vi "Add Item Buffered.vi"(6 "Items Array Length":i32=5, 8 "错误输入":errorcluster, 10 "Item":string, 11 "Listbox Ref":refnum<vi>) -> (0 "错误输出":errorcluster, 3 "Dup Listbox Ref":refnum<vi>)   [LabVIEW 2012, in "Listbox Tool.lvlib"]
uses:
  Listbox Tool.lvlib
  Custom Type/Read and Write Mode.ctl
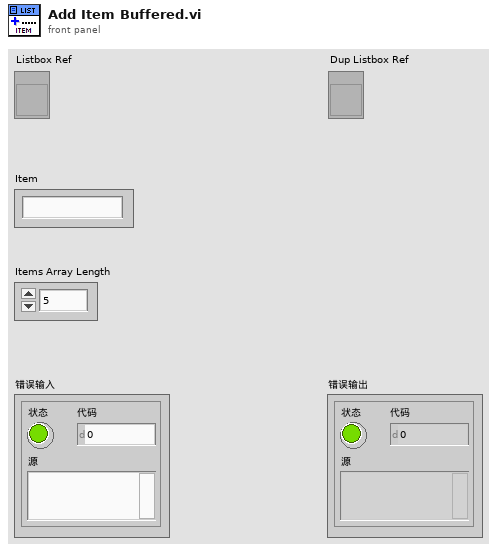
[diagram p1: front panel]
types:
  T1 = typedef "Listbox Tool.lvlib/Read and Write Mode.ctl" = enum16{"Read", "Write"}
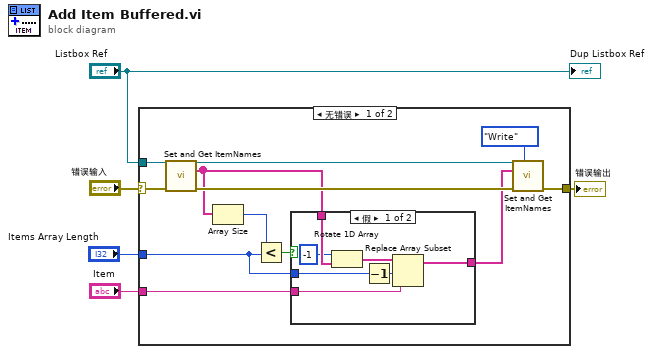
[diagram p0: block diagram]
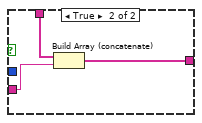
[diagram p2: hidden frame]
diagram:
  n1 = case shown="无错误" "错误输入" {
    selector: "错误输入" -> [w17 w28]
    tunnel: "Listbox Ref" -> [w16 _]
    tunnel: "Item" -> [w8 _]
    tunnel: [w12 w28] -> w2
    tunnel: "Items Array Length" -> [w6 _]
    frame No Error {
      n2 = call "Set and Get ItemNames.vi"("错误输入"=w17, "Listbox Ref"=w16) -> ("错误输出"=w15:errorcluster, "ItemNames Out"=w9:string[], "Dup Listbox Ref"=w14:refnum<vi>)  [unwired: 7 in]
      n3 = Array Size(array=w9) -> (size(s)=w11:i32)
      n4 = Less?(x=w11, y=w6) -> (x < y?=w10:bool)
      n5 = case shown="假" w10 {
        tunnel: w9 -> [w24 w27]
        tunnel: w8 -> [w21 w26]
        tunnel: [w20 w25] -> w7
        tunnel: w6 -> [w18 _]
        frame False {
          n6 = Rotate 1D Array(1:w24, 2:-1 ("n")) -> (0:w22:string[])
          n7 = Decrement(x=w18) -> (x-1=w19:i32)
          n8 = Replace Array Subset(array=w22, new element=w21, index=w19) -> (w20:string[])
        }
        frame True {
          n9 = Build Array (concatenate)(w27, w26) -> (w25:string[])
        }
      }
      n10 = call "Set and Get ItemNames.vi"("Mode"=Read_and_Write_Mode."Write", "错误输入"=w15, "ItemNames In"=w7, "Listbox Ref"=w14) -> ("错误输出"=w12:errorcluster)  [unwired: 5 in, 2 out]
    }
    frame Error {
    }
  }
  "错误输出" <- w2
  "Dup Listbox Ref" <- "Listbox Ref"
